vi "Application Name--constant.vi"() -> (3 "Application Name":string)   [LabVIEW 2019, in "Application.lvlib"]
doc: "Return the Application name.\n_____\nBased on Delacor QMH Project Template 5.0.0.82."
uses:
  Application.lvlib
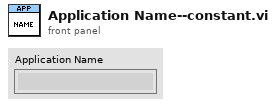
[diagram p1: front panel]
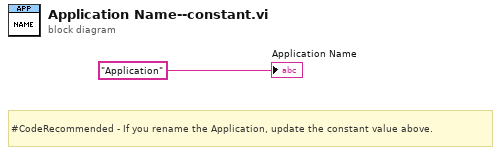
[diagram p0: block diagram]
diagram:
  # "#CodeRecommended - If you rename the Application, update the constant value above."
  "Application Name" <- "Application" ("Application Name 2")
